vi "Manager.vi"(8 "Error In":errorcluster, 11 "Shared Library In":path=path "") -> (0 "Error Out":errorcluster, 3 "Shared Library Out":path)   [LabVIEW 2017, in "LabSSH2.lvlib"]
uses:
  LabSSH2.lvlib
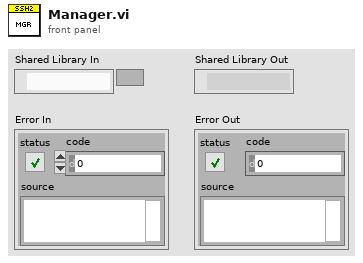
[diagram p1: front panel]
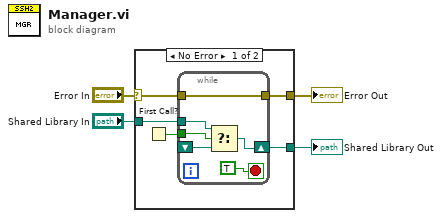
[diagram p0: block diagram]
diagram:
  n1 = case shown="No Error" "Error In" {
    selector: "Error In" -> [w9 w16]
    tunnel: [w5 w16] -> w3
    tunnel: [w7 _] -> w2
    tunnel: "Shared Library In" -> [w6 _]
    frame No Error {
      n2 = First Call?() -> (First Call?: T/F=w8:bool)
      n3 = while {
        tunnel: w9 -> [w10]
        tunnel: w8 -> [w14]
        shift-right: [w12] -> w7
        shift-left: _ -> [w11]
        tunnel: w6 -> [w13]
        tunnel: [w10] -> w5
        stop <- TRUE stop-if-true
        n4 = Select(t=w13, s=w14, f=w11) -> (s? t:f=w12:path)
      }
    }
    frame Error {
    }
  }
  "Error Out" <- w3
  "Shared Library Out" <- w2
